vi "Формирование слова данных (SubVI).vi"(11 "Data":u16) -> (3 "СД":bool[](array[boolean]))   [LabVIEW 2015]
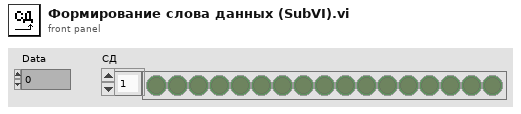
[diagram p1: front panel]
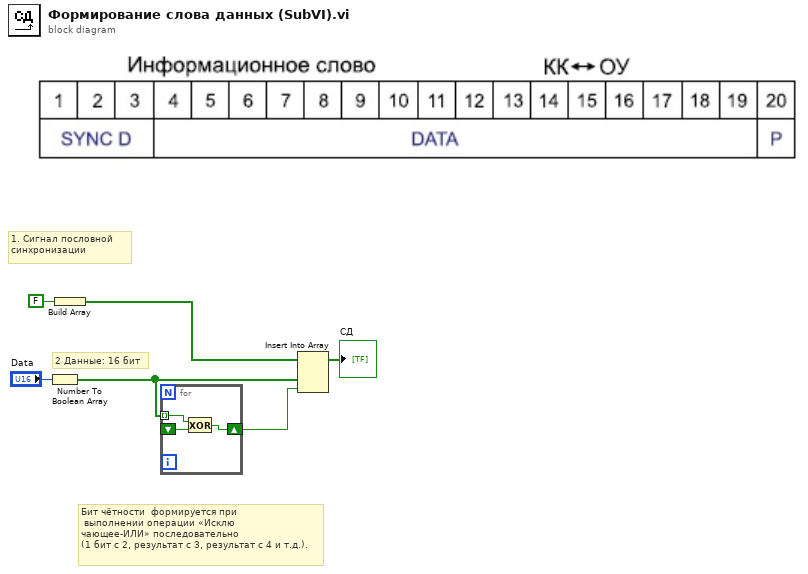
[diagram p0: block diagram]
diagram:
  # "2 Данные: 16 бит"
  # "Бит чётности  формируется при\n выполнении операции «Исклю\nчающее-ИЛИ» последовательно \n(1 бит с 2, результат с 3, результат с 4 и т.д.)."
  # "1. Сигнал пословной \nсинхронизации"
  n1 = Number To Boolean Array(number="Data") -> (Boolean array=w5:bool[])
  n2 = Build Array(FALSE) -> (w1:bool[])
  n3 = for {
    tunnel: w5 -> [w9] mode=indexing
    shift-right: [w8] -> w6
    shift-left: _ -> [w7]
    n4 = Exclusive Or(1:w7, 2:w9) -> (0:w8:bool)
  }
  n5 = Insert Into Array(array=w1, new element #1=w5, new element #2=w6) -> (→"СД":bool[])  [unwired: 1 in]
